vi "TSM DAQmx Relay Control Per-Site.vi"(0 "TSM DAQmx Relay In":T1, 2 "Settling Time (s)":dbl, 5 "Per-Site Relay Actions":T3[](array[typedef]) items=["Open Relay"=20, "Close Relay"=21], 11 "error in":errorcluster) -> (15 "error out":errorcluster)   [LabVIEW 2019]
doc: "Performs the specified per-site relay actions on all specified relays. \n\n-If the action array has one element the function maps it to all sites\n-If the array is an even multiple size of the number of sites it maps the array multiple times (used to expand across sites)\n-If the action array is not an even multiple size the function maps the array and emits a warning\n-If the action array is larger than the sites it gets shortened and the function emits a warning"
uses:
  <vilib>/NI_TestStand_SemiconductorModule/NI_TestStand_Semiconductor_Module.lvlibp/1abvi3w/instr.lib/niSwitch/niswitch.llb/niSwitch Relay Action.ctl
  Pin Map/TSM DAQmx Relay.ctl
  <vilib>/NI_TestStand_SemiconductorModule/NI_TestStand_Semiconductor_Module.lvlibp/PinMap/General/SemiconductorModuleContext.ctl
  ee22f031-ec38-4f28-81b6-ff4c7fb4bdad.vi
  <vilib>/Utility/error.llb/Error Cluster From Error Code.vi
  SubVIs/TSM DAQmx Relay Write.vi
  <vilib>/Utility/High Resolution Polling Wait.vi
  <vilib>/NI_TestStand_SemiconductorModule/NI_TestStand_Semiconductor_Module.lvlibp
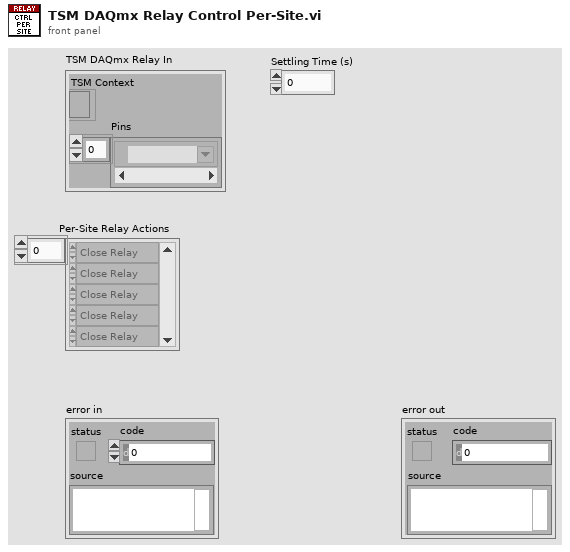
[diagram p1: front panel]
types:
  T1 = typedef "TSM DAQmx Relay.ctl" = cluster{"TSM Context":T2, "Pins":tag[]}
  T2 = typedef "NI_TestStand_Semiconductor_Module.lvlibp/SemiconductorModuleContext.ctl" = refnum<k7>
  T3 = typedef "NI_TestStand_Semiconductor_Module.lvlibp/niSwitch Relay Action.ctl" = i32
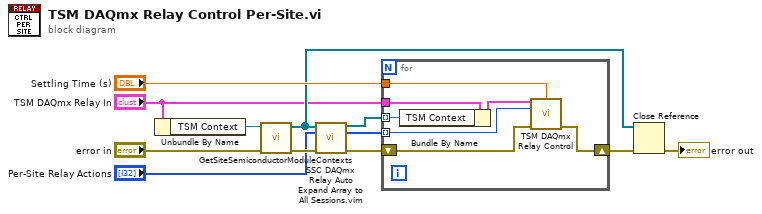
[diagram p0: block diagram]
diagram:
  n1 = Unbundle By Name("TSM DAQmx Relay In") -> ("TSM Context"=w10:T2)
  n2 = call <vilib>:"GetSiteSemiconductorModuleContexts.vi"("error in (no error)"="error in", "Semiconductor Module Context"=w10) -> ("error out"=w9:errorcluster, "Site Semiconductor Module Contexts"=w2:T2[])  [unwired: 8 in]
  n3 = call "SSC DAQmx Relay Auto Expand Array to All Sessions.vim"("Relay TSM In"=w2, "Data In"="Per-Site Relay Actions", "error in"=w9) -> ("Relay TSM Out"=w3:T2[], "Data Out"=w7:T3[], "error out"=w5:errorcluster)  [unwired: 10 in]
  n4 = for {
    tunnel: "Settling Time (s)" -> [w13]
    tunnel: w7 -> [w16] mode=indexing
    shift-right: [w14] -> w6
    shift-left: w5 -> [w19]
    tunnel: w3 -> [w15] mode=indexing
    tunnel: "TSM DAQmx Relay In" -> [w18]
    n5 = Bundle By Name(cluster=w18, "TSM Context"=w15) -> (w17:T1)
    n6 = call "TSM DAQmx Relay Control.vi"("TSM DAQmx Relay In"=w17, "Settling Time (s)"=w13, "Relay Action"=w16, "error in"=w19) -> ("error out"=w14:errorcluster)  [unwired: 11 in]
  }
  n7 = Close Reference(reference=w2, error in (no error)=w6) -> (error out=→"error out":errorcluster)
